vi "KH TURCK ETHERNETIP RFID Status.vi"(6 "Nr.Module":i32, 8 "RFID 1":T1={"NumberOfBytes"=112, "State"="", "Counter"=0, "ReadData"=[], "AnzahlFragmente"=0, "WritingFinished"=FALSE, "ReadingFinished"=FALSE, "UID"=[], "ActCommand"=enum."Inventory", "SizeFragmentRead"=112, "LengthUID"=112, "WriteDataInclUID"=[], "Timeout"=FALSE, "SizeFragmentWrite"=112}, 11 "RFID 0":T1={"NumberOfBytes"=112, "State"="", "Counter"=0, "ReadData"=[], "AnzahlFragmente"=0, "WritingFinished"=FALSE, "ReadingFinished"=FALSE, "UID"=[], "ActCommand"=enum."Inventory", "SizeFragmentRead"=112, "LengthUID"=112, "WriteDataInclUID"=[], "Timeout"=FALSE, "SizeFragmentWrite"=112}) -> (3 "StatusOUT":T3)   [LabVIEW 2021]
uses:
  KH TURCK ETHERNETIP TDefCluster TBEN-S2-2RFID-4DXP Status.ctl
  KH TURCK ETHERNETIP TDefCluster TURCK RFID.ctl
  KH TURCK ETHERNETIP TDef Enum RFID Act Command.ctl
  KH TURCK ETHERNETIP RFID Global.vi
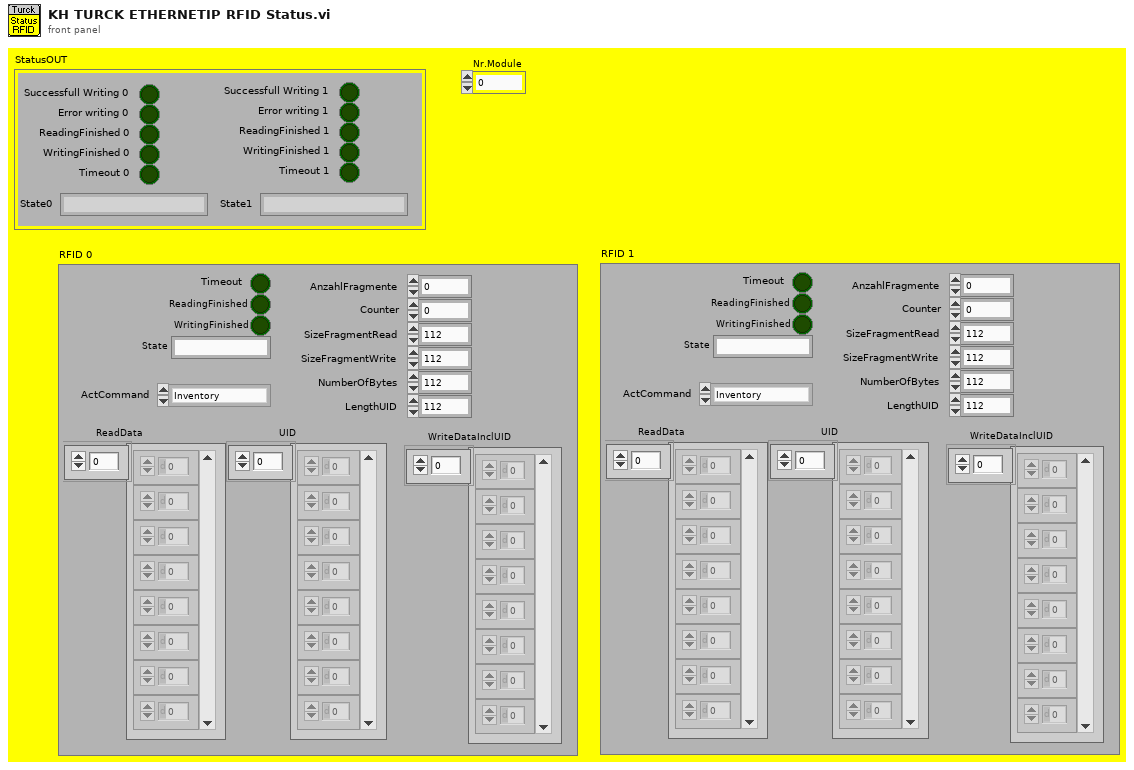
[diagram p1: front panel]
types:
  T1 = typedef "KH TURCK ETHERNETIP TDefCluster TURCK RFID.ctl" = cluster{"NumberOfBytes":i32, "State":string, "Counter":i32, "ReadData":u8[], "AnzahlFragmente":i32, "WritingFinished":bool, "ReadingFinished":bool, "UID":u8[], "ActCommand":T2, "SizeFragmentRead":i32, "LengthUID":u16, "WriteDataInclUID":u8[], "Timeout":bool, "SizeFragmentWrite":i32}
  T2 = typedef "KH TURCK ETHERNETIP TDef Enum RFID Act Command.ctl" = enum16{"read", "write", "idle", "Inventory", ""}
  T3 = typedef "KH TURCK ETHERNETIP TDefCluster TBEN-S2-2RFID-4DXP Status.ctl" = cluster{"Error writing 1":bool, "ReadingFinished 1":bool, "WritingFinished 1":bool, "Error writing 0":bool, "ReadingFinished 0":bool, "WritingFinished 0":bool, "Timeout 1":bool, "State0":string, "State1":string, "Timeout 0":bool, "Successfull Writing 1":bool, "Successfull Writing 0":bool}
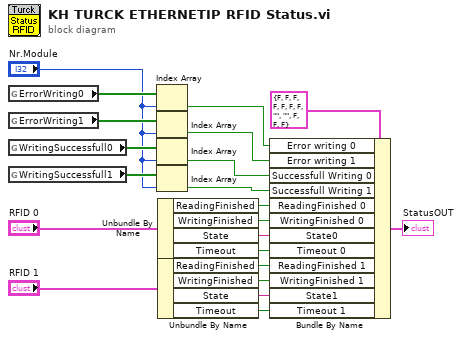
[diagram p0: block diagram]
diagram:
  n1 = global read "KH TURCK ETHERNETIP RFID Global.vi" "ErrorWriting0"() -> (w5:bool[])
  n2 = global read "KH TURCK ETHERNETIP RFID Global.vi" "ErrorWriting1"() -> (w6:bool[])
  n3 = global read "KH TURCK ETHERNETIP RFID Global.vi" "WritingSuccessfull0"() -> (w7:bool[])
  n4 = global read "KH TURCK ETHERNETIP RFID Global.vi" "WritingSuccessfull1"() -> (w9:bool[])
  n5 = Index Array(array=w5, index="Nr.Module") -> (element=w1:bool)
  n6 = Index Array(array=w6, index="Nr.Module") -> (element=w2:bool)
  n7 = Index Array(array=w7, index="Nr.Module") -> (element=w3:bool)
  n8 = Index Array(array=w9, index="Nr.Module") -> (element=w8:bool)
  n9 = Unbundle By Name("RFID 0") -> ("ReadingFinished"=w19:bool, "WritingFinished"=w18:bool, "State"=w17:string, "Timeout"=w16:bool)
  n10 = Unbundle By Name("RFID 1") -> ("ReadingFinished"=w14:bool, "WritingFinished"=w13:bool, "State"=w12:string, "Timeout"=w11:bool)
  n11 = Bundle By Name(cluster=T3 {"Error writing 1"=FALSE, "ReadingFinished 1"=FALSE, "WritingFinished 1"=FALSE, "Error writing 0"=FALSE, "ReadingFinished 0"=FALSE, "WritingFinished 0"=FALSE, "Timeout 1"=FALSE, "State0"="", "State1"="", "Timeout 0"=FALSE, "Successfull Writing 1"=FALSE, "Successfull Writing 0"=FALSE} ("StatusOUT 2"), "Error writing 0"=w1, "Error writing 1"=w2, "Successfull Writing 0"=w3, "Successfull Writing 1"=w8, "ReadingFinished 0"=w19, "WritingFinished 0"=w18, "State0"=w17, "Timeout 0"=w16, "ReadingFinished 1"=w14, "WritingFinished 1"=w13, "State1"=w12, "Timeout 1"=w11) -> (→"StatusOUT":T3)
